vi "Cash Karp Check.vi"(8 "F(X,t)":string[](array[string]), 9 "X":string[](array[string]), 10 "time":string, 11 "X(0)":dbl[](array[numeric]) format="%.2f") -> (0 "system OK":bool, 1 "error text":string[](array[string]), 2 "error":i32[](array[numeric]), 3 "error message":string, 4 "zero array":dbl[](array[numeric]), 5 "result":dbl[][](array[numeric]), 7 "table":i32[][][](array[numeric]))   [LabVIEW 2017, in "NI_Gmath.lvlib"]
uses:
  NI_Gmath.lvlib
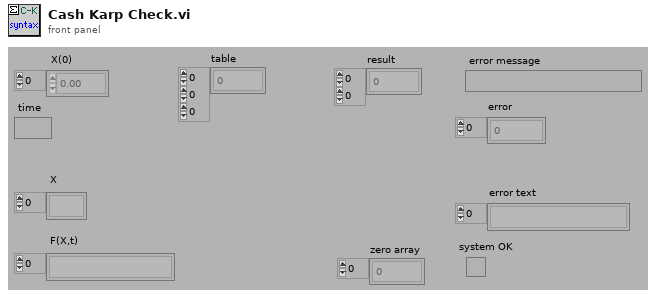
[diagram p1: front panel]
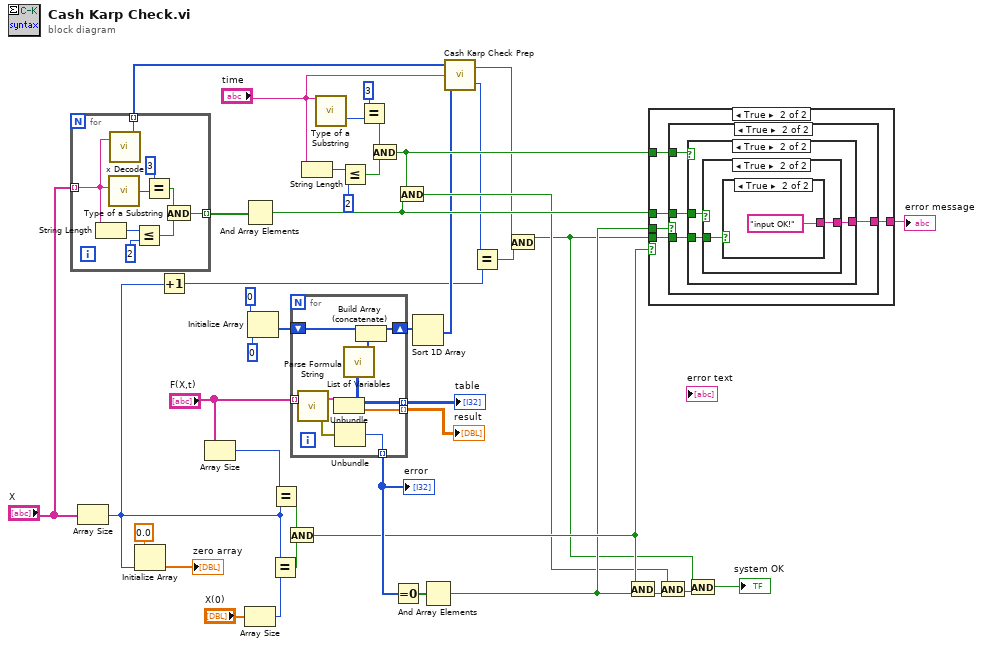
[diagram p0: block diagram]
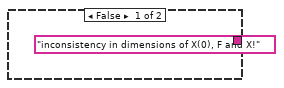
[diagram p2: hidden frame]
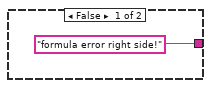
[diagram p3: hidden frame]
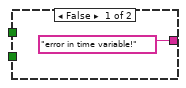
[diagram p4: hidden frame]
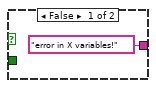
[diagram p5: hidden frame]
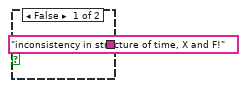
[diagram p6: hidden frame]
diagram:
  n1 = for {
    tunnel: "X" -> [w44] mode=indexing
    tunnel: [w45] -> w23 mode=indexing
    tunnel: [w43] -> w14 mode=indexing
    n2 = String Length(string=w44) -> (length=w46:i32)
    n3 = call "Type of a Substring.VI"("item"=w44) -> ("type"=w48:i32)
    n4 = call "x Decode.vi"("x string"=w44) -> ("number"=w43:i32)  [unwired: 1 in, 1 out]
    n5 = Less Or Equal?(x=w46, y=2) -> (x <= y?=w50:bool)
    n6 = Equal?(x=3, y=w48) -> (x = y?=w51:bool)
    n7 = And(x=w51, y=w50) -> (x .and. y?=w45:bool)
  }
  n8 = Array Size(array="X") -> (size(s)=w3:i32)
  n9 = Initialize Array(0.0, w3) -> (→"zero array":dbl[])
  n10 = Increment(x=w3) -> (x+1=w13:i32)
  n11 = Array Size(array="F(X,t)") -> (size(s)=w37:i32)
  n12 = And Array Elements(Boolean array=w23) -> (logical AND=w21:bool)
  n13 = Array Size(array="X(0)") -> (size(s)=w36:i32)
  n14 = Initialize Array(0, 0) -> (w17:i32[])
  n15 = Equal?(x=w3, y=w36) -> (x = y?=w35:bool)
  n16 = Equal?(x=w37, y=w3) -> (x = y?=w34:bool)
  n17 = And(x=w34, y=w35) -> (x .and. y?=w33:bool)
  n18 = for {
    tunnel: [w55] -> w41 mode=indexing
    tunnel: [w53] -> w40 mode=indexing
    tunnel: [w52] -> w39 mode=indexing
    tunnel: "F(X,t)" -> [w60] mode=indexing
    shift-right: [w58] -> w16
    shift-left: w17 -> [w59]
    n19 = call "Parse Formula String.vi"("formula"=w60) -> ("error out"=w56:errorcluster, "Parsed Formula"=w54:cluster{"Table":i32[][], "Y Values":dbl[]})  [unwired: 1 in]
    n20 = Unbundle(w54) -> ("Table"=w53:i32[][], "Y Values"=w52:dbl[])
    n21 = Unbundle(w56) -> ("code"=w55:i32)  [unwired: 2 out]
    n22 = call "List of Variables.vi"("Table"=w53) -> ("List of variables"=w57:i32[])
    n23 = Build Array (concatenate)(w59, w57) -> (w58:i32[])
  }
  "error" <- w41
  "result" <- w39
  "table" <- w40
  n24 = String Length(string="time") -> (length=w30:i32)
  n25 = call "Type of a Substring.VI"("item"="time") -> ("type"=w28:i32)
  n26 = Less Or Equal?(x=w30, y=2) -> (x <= y?=w26:bool)
  n27 = Equal?(x=3, y=w28) -> (x = y?=w25:bool)
  n28 = And(x=w25, y=w26) -> (x .and. y?=w22:bool)
  n29 = Equal To 0?(x=w41) -> (x = 0?=w42:bool[])
  n30 = And(x=w22, y=w21) -> (x .and. y?=w20:bool)
  n31 = Sort 1D Array(array=w16) -> (sorted array=w15:i32[])
  n32 = And Array Elements(Boolean array=w42) -> (logical AND=w31:bool)
  n33 = call "Cash Karp Check Prep.vi"("F(X,t) coded"=w15, "time"="time", "X coded"=w14) -> ("number of X variables"=w12:i32, "variables correct?"=w4:bool)
  n34 = Equal?(x=w12, y=w13) -> (x = y?=w11:bool)
  n35 = And(x=w4, y=w11) -> (x .and. y?=w10:bool)
  n36 = And(x=w33, y=w31) -> (x .and. y?=w24:bool)
  n37 = case shown="True" w33 {
    tunnel: ["inconsistency in dimensions of X(0), F and X!" w66] -> w32
    tunnel: w31 -> [_ w65]
    tunnel: w21 -> [_ w64]
    tunnel: w22 -> [_ w63]
    tunnel: w10 -> [_ w62]
    frame False {
    }
    frame True {
      n38 = case shown="True" w65 {
        tunnel: ["formula error right side!" w71] -> w66
        tunnel: w64 -> [_ w70]
        tunnel: w63 -> [_ w69]
        tunnel: w62 -> [_ w68]
        frame False {
        }
        frame True {
          n39 = case shown="True" w69 {
            tunnel: ["error in time variable!" w75] -> w71
            tunnel: w70 -> [_ w74]
            tunnel: w68 -> [_ w73]
            frame False {
            }
            frame True {
              n40 = case shown="True" w74 {
                tunnel: ["error in X variables!" w78] -> w75
                tunnel: w73 -> [_ w77]
                frame False {
                }
                frame True {
                  n41 = case shown="True" w77 {
                    tunnel: ["inconsistency in structure of time, X and F!" "input OK!"] -> w78
                    frame False {
                    }
                    frame True {
                    }
                  }
                }
              }
            }
          }
        }
      }
    }
  }
  "error message" <- w32
  n42 = And(x=w20, y=w24) -> (x .and. y?=w9:bool)
  n43 = And(x=w10, y=w9) -> (x .and. y?=→"system OK":bool)
